vi "credential check_19-07-16.vi"(8 "error in":errorcluster, 9 "PASSWORD":string, 10 "USER NAME":string, 11 "file path (dialog if empty)":path) -> (0 "error out":errorcluster, 2 "USER EXISTS?":bool, 3 "user?":string)   [LabVIEW 2019, in "ZenGage v3.0 UI.lvclass"]
uses:
  ZenGage v3.0 UI.lvclass
  <vilib>/Utility/file.llb/Read Delimited Spreadsheet (string).vi
panel:
  in  "appended path":path
  out "all rows":string[][](array[string])
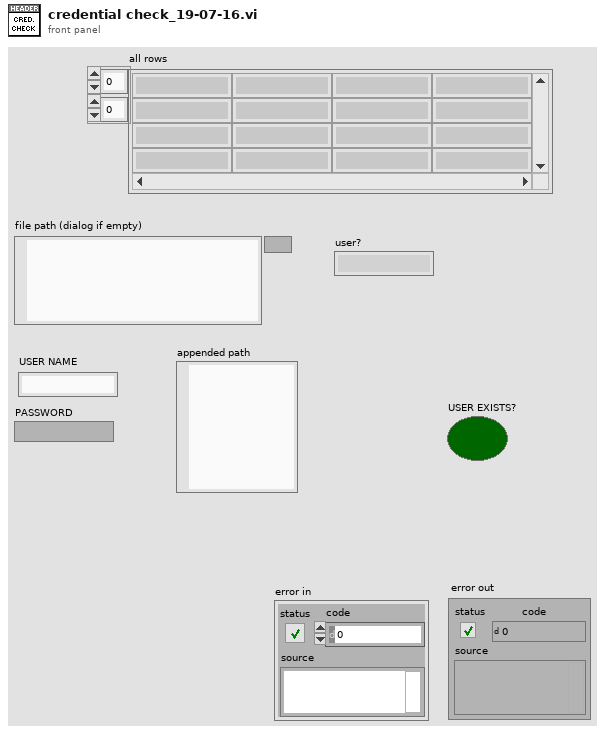
[diagram p1: front panel]
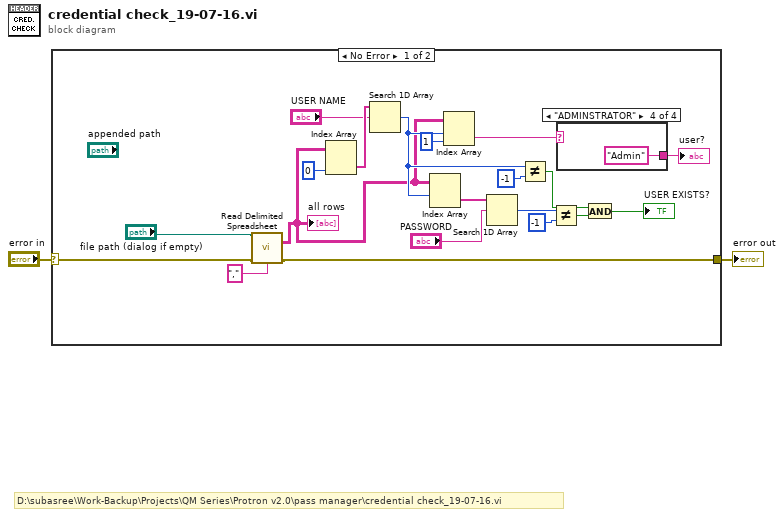
[diagram p0: block diagram]
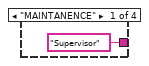
[diagram p2: hidden frame]
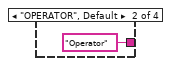
[diagram p3: hidden frame]
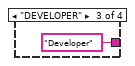
[diagram p4: hidden frame]
diagram:
  # "D:\\subasree\\Work-Backup\\Projects\\QM Series\\Protron v2.0\\pass manager\\credential check_19-07-16.vi"
  n1 = case shown="No Error" "error in" {
    selector: "error in" -> [w7 w27]
    tunnel: [w6 w27] -> w2
    frame No Error {
      n2 = call-poly <vilib>:"Read Delimited Spreadsheet.vi"("file path (dialog if empty)"="file path (dialog if empty)", "error in (no error)"=w7, "delimiter (\\t)"="," ("delimiter (\\t)")) -> ("all rows"=w4:string[][], "error out"=w6:errorcluster)  [unwired: 7 in, 4 out]
      "all rows" <- w4
      n3 = Index Array(array=w4, index (col)=0 ("disabled index (col)")) -> (element=w21:string[])  [unwired: 1 in]
      n4 = Search 1D Array(1D array=w21, element="USER NAME") -> (index of element=w12:i32)  [unwired: 1 in]
      n5 = Index Array(array=w4, index (row)=w12) -> (element=w15:string[])  [unwired: 1 in]
      n6 = Index Array(array=w4, index (row)=w12, index (col)=1 ("disabled index (col)")) -> (element=w10:string)
      n7 = Search 1D Array(1D array=w15, element="PASSWORD") -> (index of element=w14:i32)  [unwired: 1 in]
      n8 = Not Equal?(x=w12, y=-1) -> (x != y?=w17:bool)
      n9 = Not Equal?(x=w14, y=-1) -> (x != y?=w16:bool)
      n10 = case shown="\"ADMINSTRATOR\"" w10 {
        tunnel: ["Supervisor" "Operator" "Developer" "Admin"] -> w9
        frame "MAINTANENCE" {
        }
        frame "OPERATOR", Default {
        }
        frame "DEVELOPER" {
        }
        frame "ADMINSTRATOR" {
        }
      }
      "user?" <- w9
      n11 = And(x=w17, y=w16) -> (x .and. y?=→"USER EXISTS?":bool)
    }
    frame Error {
    }
  }
  "error out" <- w2
